vi "USB2XXX_LINEX_MLXProgramer.vi"() -> ()   [LabVIEW 2010]
panel:
  in  "Use Fast LIN":u8(ring) items=["LIN", "Fast LIN"]
  in  "Loader File Name":string="loaderB-81108_9C-lin2x-19200-loader.hex"
  in  "App File Name":string
  out "Result":bool
  in  "BaudRateOfKbps":u8=20
  in  "Channel Index":u8(ring) items=["LIN1", "LIN2"]
  in  "Device Index":i32(ring) items=["0", "1", "2", "3", "4", "5"]
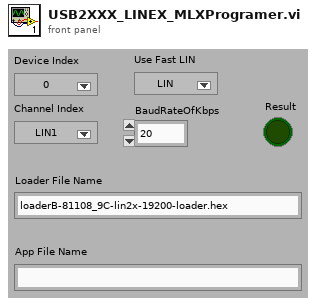
[diagram p1: front panel]
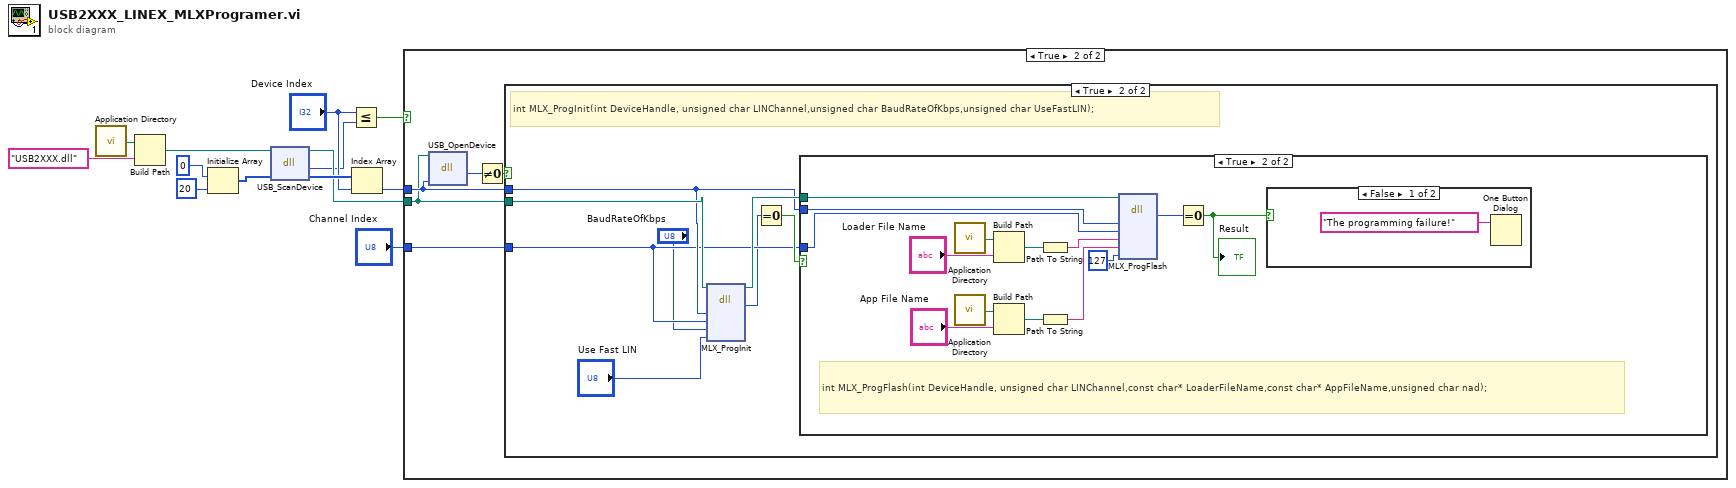
[diagram p0: block diagram]
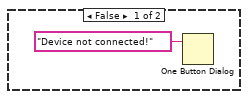
[diagram p2: hidden frame]
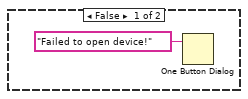
[diagram p3: hidden frame]
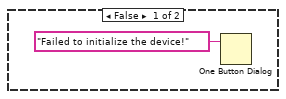
[diagram p4: hidden frame]
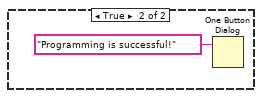
[diagram p5: hidden frame]
diagram:
  n1 = call <vilib>:"Application Directory.vi"() -> ("Application Directory"=w6:path)
  n2 = Build Path(base path=w6, name or relative path="USB2XXX.dll") -> (appended path=w5:path)
  n3 = Initialize Array(0, 20 ("dimension size")) -> (w10:i32[])
  n4 = dll-call lib="E:/OtherWork/STM32/USB2XXX_Example/examples/Labview/PublicFiles/USB2XXX.dll" fn="USB_ScanDevice"(path in=w5, "pDevNum"=w10) -> (path out=w8:path, "return type"=w2:i32, "pDevNum"=w13:i32[])  [unwired: 2 in, 1 out]
  n5 = Less Or Equal?(x="Device Index", y=w2) -> (x <= y?=w4:bool)
  n6 = Index Array(array=w13, index="Device Index") -> (element=w9:i32)
  n7 = case shown="True" w4 {
    tunnel: w9 -> [_ w17]
    tunnel: w8 -> [_ w16]
    tunnel: "Channel Index" -> [_ w15]
    frame False {
      n8 = One Button Dialog(message="Device not connected!") -> ()  [unwired: 1 in, 1 out]
    }
    frame True {
      n9 = dll-call lib="E:/OtherWork/STM32/USB2XXX_Example/examples/Labview/PublicFiles/USB2XXX.dll" fn="USB_OpenDevice"(path in=w16, "DevIndex"=w17) -> ("return type"=w19:u8)  [unwired: 3 in, 2 out]
      n10 = Not Equal To 0?(x=w19) -> (x != 0?=w18:bool)
      n11 = case shown="True" w18 {
        tunnel: w17 -> [_ w25]
        tunnel: w16 -> [_ w27]
        tunnel: w15 -> [_ w24]
        frame False {
          n12 = One Button Dialog(message="Failed to open device!") -> ()  [unwired: 1 in, 1 out]
        }
        frame True {
          # "int MLX_ProgInit(int DeviceHandle, unsigned char LINChannel,unsigned char BaudRateOfKbps,unsigned char UseFastLIN);"
          n13 = dll-call lib="E:/Projects/USB2XXX/trunk/USB2XXX/USB2XXX/vs2010/Release/USB2XXX.*" fn="MLX_ProgInit"(path in=w27, "DeviceHandle"=w25, "LINChannel"=w24, "BaudRateOfKbps"="BaudRateOfKbps", "UseFastLIN"="Use Fast LIN") -> (path out=w26:path, "return type"=w21:i32)  [unwired: 6 in, 1 out]
          n14 = Equal To 0?(x=w21) -> (x = 0?=w28:bool)
          n15 = case shown="True" w28 {
            tunnel: w24 -> [_ w41]
            tunnel: w25 -> [_ w42]
            tunnel: w26 -> [_ w43]
            frame False {
              n16 = One Button Dialog(message="Failed to initialize the device!") -> ()  [unwired: 1 in, 1 out]
            }
            frame True {
              # "int MLX_ProgFlash(int DeviceHandle, unsigned char LINChannel,const char* LoaderFileName,const char* AppFileName,unsigned char nad);"
              n17 = call <vilib>:"Application Directory.vi"() -> ("Application Directory"=w38:path)
              n18 = call <vilib>:"Application Directory.vi"() -> ("Application Directory"=w39:path)
              n19 = Build Path(base path=w38, name or relative path="Loader File Name") -> (appended path=w37:path)
              n20 = Build Path(base path=w39, name or relative path="App File Name") -> (appended path=w36:path)
              n21 = Path To String(path=w37) -> (string=w35:string)
              n22 = Path To String(path=w36) -> (string=w34:string)
              n23 = dll-call lib="E:/Projects/USB2XXX/trunk/USB2XXX/USB2XXX/vs2010/Release/USB2XXX.*" fn="MLX_ProgFlash"(path in=w43, "DeviceHandle"=w42, "LINChannel"=w41, "LoaderFileName"=w35, "AppFileName"=w34, "nad"=u8 127) -> ("return type"=w33:i32)  [unwired: 7 in, 2 out]
              n24 = Equal To 0?(x=w33) -> (x = 0?=w32:bool)
              "Result" <- w32
              n25 = case shown="False" w32 {
                frame False {
                  n26 = One Button Dialog(message="The programming failure!") -> ()  [unwired: 1 in, 1 out]
                }
                frame True {
                  n27 = One Button Dialog(message="Programming is successful!") -> ()  [unwired: 1 in, 1 out]
                }
              }
            }
          }
        }
      }
    }
  }
